vi "Layer1_ReceiveResponse.vi"(8 "Error In":errorcluster, 10 "Close Port After?":bool=TRUE, 11 "Serial Port to Use (In)":refnum<visa-resource-name>="COM8") -> (0 "Error Out":errorcluster, 1 "Layer1 Payload":string, 2 "Layer 1 Valid Packet":bool, 3 "Serial Port to Use (out)":refnum<visa-resource-name>, 5 "Raw Rx byte array":u8[](array[numeric]), 7 "Raw Receive Buffer":string)   [LabVIEW 2012]
uses:
  Arduino_Serial_GlobalConstants.vi
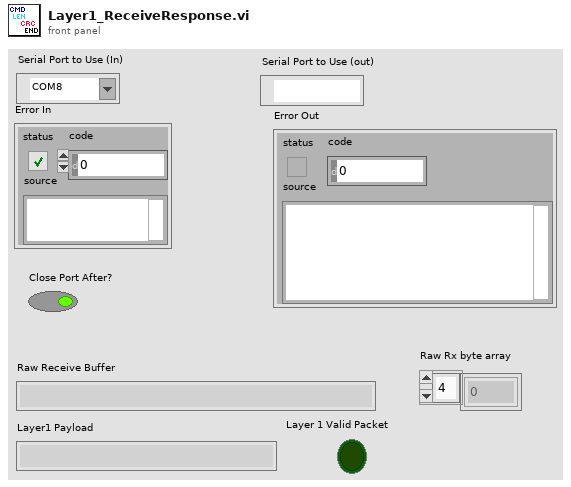
[diagram p1: front panel]
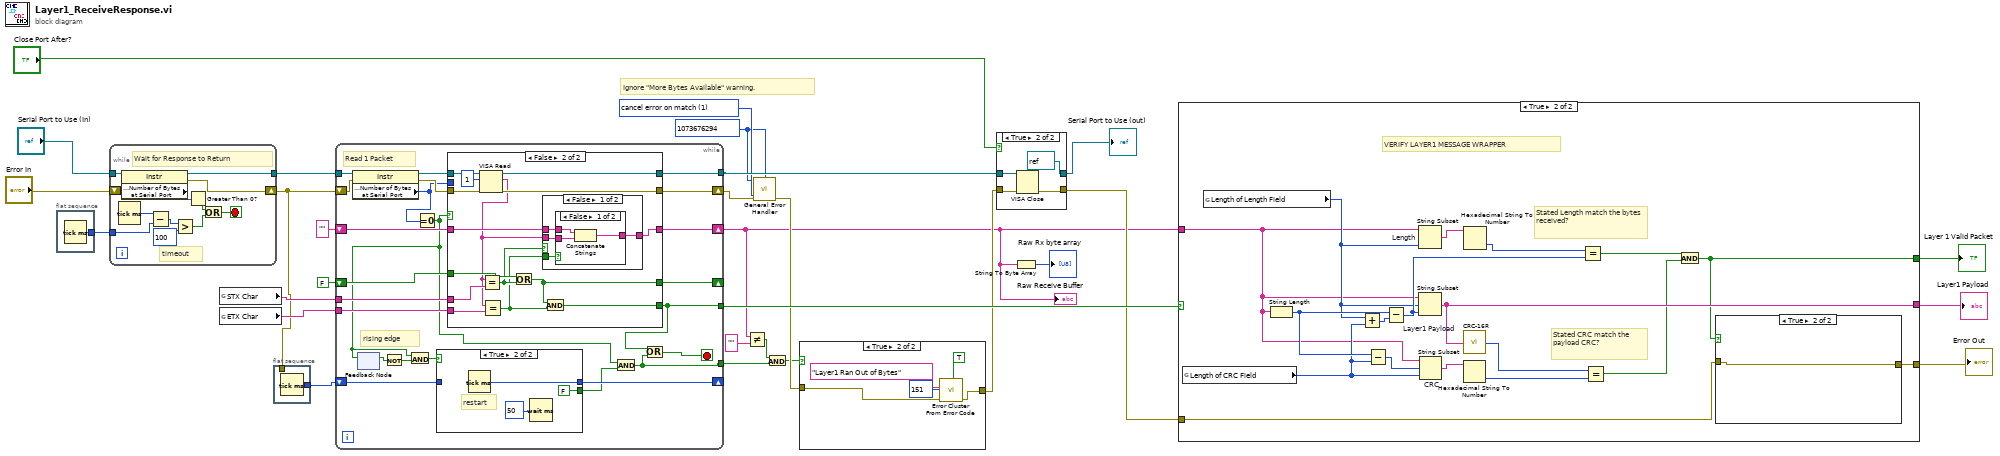
[diagram p0: block diagram]
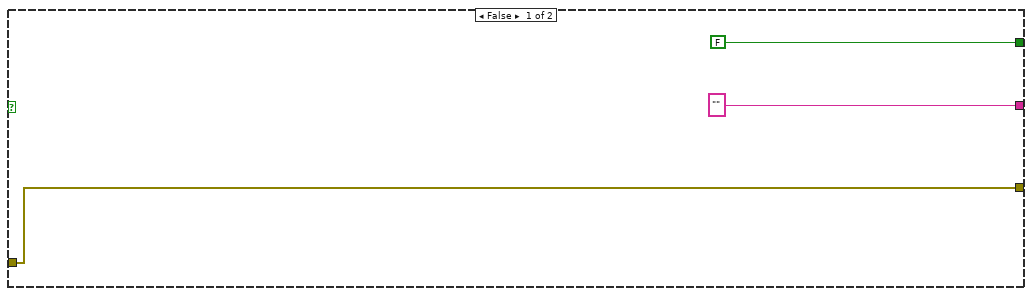
[diagram p4: hidden frame]
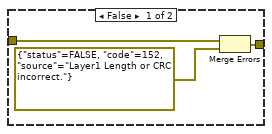
[diagram p5: hidden frame]
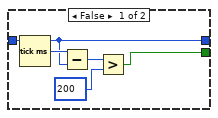
[diagram p6: hidden frame]
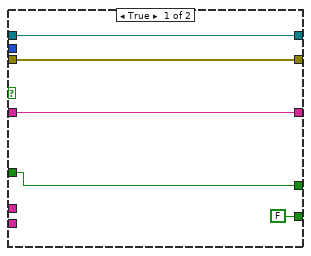
[diagram p7: hidden frame]
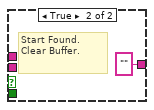
[diagram p9: hidden frame]
diagram:
  w8 = 1073676294 ("[exception code]")
  w9 = 1 items=["no exception", "cancel error on match", "set error on match"] ("[exception action] (none:0)")
  # "Ignore \"More Bytes Available\" warning."
  n1 = flat-sequence {
    tunnel: [w30] -> w22
    frame #0 {
      n2 = Tick Count (ms)() -> (millisecond timer value=w30:u32)
    }
  }
  n3 = while {
    tunnel: "Serial Port to Use (In)" -> [w42]
    shift-right: [w32] -> w13
    shift-left: "Error In" -> [w41]
    tunnel: w22 -> [w39]
    tunnel: [w33] -> w28
    stop <- w34 stop-if-true
    # "Wait for Response to Return"
    # "timeout"
    n4 = Tick Count (ms)() -> (millisecond timer value=w40:u32)
    n5 = property class="Instr"(reference=w42, error in=w41) -> (reference out=w33:refnum<visa-resource-name>, error out=w32:errorcluster, "Serial Settings:Number of Bytes at Serial Port"=w31:u32)
    n6 = Subtract(x=w40, y=w39) -> (x-y=w38:u32)
    n7 = Greater?(x=w38, y=u32 100) -> (0:w36:bool)
    n8 = Greater Than 0?(x=w31) -> (x > 0?=w35:bool)
    n9 = Or(x=w35, y=w36) -> (x .or. y?=w34:bool)
  }
  n10 = global read "Arduino_Serial_GlobalConstants.vi" "STX Char"() -> (w24:string)
  n11 = global read "Arduino_Serial_GlobalConstants.vi" "ETX Char"() -> (w23:string)
  n12 = flat-sequence {
    tunnel: [w43] -> w14
    tunnel: w13 -> [_]
    frame #0 {
      n13 = Tick Count (ms)() -> (millisecond timer value=w43:u32)
    }
  }
  n14 = while {
    tunnel: w28 -> [w66]
    shift-right: [w63] -> w7
    shift-left: w13 -> [w65]
    tunnel: [w62] -> w26
    shift-right: [w61] -> w5
    shift-left: "" -> [w60]
    tunnel: w24 -> [w57]
    tunnel: w23 -> [w56]
    shift-right: [w49] -> _
    shift-left: w14 -> [w50]
    shift-right: [w55] -> _
    shift-left: FALSE -> [w54]
    tunnel: [w52] -> w17
    tunnel: [w51] -> w1
    stop <- w53 stop-if-true
    # "rising edge"
    # "Read 1 Packet"
    n15 = property class="Instr"(reference=w66, error in=w65) -> (reference out=w64:refnum<visa-resource-name>, error out=w59:errorcluster, "Serial Settings:Number of Bytes at Serial Port"=w58:u32)
    n16 = feedback #1() -> (w44:bool)  [unwired: 1 in]
    n17 = Not(x=w44) -> (.not. x?=w45:bool)
    n18 = Equal To 0?(x=w58) -> (x = 0?=w46:bool)
    n19 = feedback-in #1(w46) -> ()
    n20 = And(x=w46, y=w45) -> (x .and. y?=w47:bool)
    n21 = case shown="True" w47 {
      tunnel: [w68 w74] -> w49
      tunnel: [w69 FALSE] -> w48
      tunnel: w50 -> [w68 _]
      frame False {
        n22 = Tick Count (ms)() -> (millisecond timer value=w71:u32)
        n23 = Subtract(x=w71, y=w68) -> (x-y=w70:u32)
        n24 = Greater?(x=w70, y=u32 200) -> (0:w69:bool)
      }
      frame True {
        # "restart"
        n25 = Tick Count (ms)() -> (millisecond timer value=w74:u32)
        n26 = Wait (ms)(milliseconds to wait=u32 50) -> ()  [unwired: 1 out]
      }
    }
    n27 = case shown="False" w46 {
      tunnel: w64 -> [w79 w94]
      tunnel: w59 -> [w78 w93]
      tunnel: w58 -> [_ _]
      tunnel: [w78 w92] -> w63
      tunnel: [w79 w91] -> w62
      tunnel: [w77 w80] -> w61
      tunnel: w60 -> [w77 w83]
      tunnel: w57 -> [_ w89]
      tunnel: w56 -> [_ w88]
      tunnel: [w76 w87] -> w55
      tunnel: w54 -> [w76 w85]
      tunnel: [FALSE w86] -> w52
      frame True {
      }
      frame False {
        n28 = VISA Read(VISA resource name=w94, byte count=u32 1, error in (no error)=w93) -> (VISA resource name out=w91:refnum<visa-resource-name>, read buffer=w82:string, error out=w92:errorcluster)  [unwired: 1 out]
        n29 = Equal?(x=w82, y=w89) -> (x = y?=w84:bool)
        n30 = Equal?(x=w82, y=w88) -> (x = y?=w81:bool)
        n31 = Or(x=w85, y=w84) -> (x .or. y?=w87:bool)
        n32 = case shown="False" w84 {
          tunnel: [w95 ""] -> w80
          tunnel: w83 -> [w97 _]
          tunnel: w82 -> [w96 _]
          tunnel: w81 -> [w98 _]
          frame False {
            n33 = case shown="False" w98 {
              tunnel: w97 -> [w101 w102]
              tunnel: w96 -> [w100 _]
              tunnel: [w99 w102] -> w95
              frame False {
                n34 = Concatenate Strings(w101, w100) -> (w99:string)
              }
              frame True {
                # "End Byte.\nDon't add."
              }
            }
          }
          frame True {
            # "Start Found.\nClear Buffer."
          }
        }
        n35 = And(x=w87, y=w81) -> (x .and. y?=w86:bool)
      }
    }
    n36 = And(x=w46, y=w48) -> (x .and. y?=w51:bool)
    n37 = Or(x=w52, y=w51) -> (x .or. y?=w53:bool)
  }
  "Raw Receive Buffer" <- w5
  n38 = Not Equal?(x=w5, y="") -> (x != y?=w2:bool)
  n39 = call <vilib>:"General Error Handler.vi"("[error code] (0)"=w8, "error in (no error)"=w7, "[exception action] (none:0)"=w9, "[exception code]"=w8) -> ("error out"=w6:errorcluster)  [unwired: 7 in, 4 out]
  n40 = And(x=w2, y=w1) -> (x .and. y?=w3:bool)
  n41 = case shown="True" w3 {
    tunnel: w6 -> [w104 w107]
    tunnel: [w104 w108] -> w10
    frame False {
    }
    frame True {
      n42 = call <vilib>:"Error Cluster From Error Code.vi"("is warning? (False)"=TRUE, "error in (no error)"=w107, "error message (\"\")"="Layer1 Ran Out of Bytes" ("source"), "error code (0)"=151) -> ("error out"=w108:errorcluster)  [unwired: 5 in]
    }
  }
  n43 = case shown="True" "Close Port After?" {
    tunnel: w10 -> [w111 w115]
    tunnel: w26 -> [w110 w114]
    tunnel: [w111 w113] -> w12
    tunnel: [w110 refnum<visa-resource-name> refnum ("VISA resource")] -> w15
    frame False {
    }
    frame True {
      n44 = VISA Close(VISA resource name=w114, error in (no error)=w115) -> (error out=w113:errorcluster)
    }
  }
  "Serial Port to Use (out)" <- w15
  n45 = String To Byte Array(string=w5) -> (unsigned byte array=→"Raw Rx byte array":u8[])
  n46 = case shown="True" w17 {
    tunnel: ["" w127] -> w21
    tunnel: [FALSE w119] -> w20
    tunnel: w5 -> [_ w122]
    tunnel: w12 -> [w116 w121]
    tunnel: [w116 w120] -> w11
    frame False {
    }
    frame True {
      # "VERIFY LAYER1 MESSAGE WRAPPER"
      # "Stated CRC match the payload CRC?"
      # "Stated Length match the bytes received?"
      n47 = global read "Arduino_Serial_GlobalConstants.vi" "Length of CRC Field"() -> (w123:i32)
      n48 = global read "Arduino_Serial_GlobalConstants.vi" "Length of Length Field"() -> (w124:i32)
      n49 = String Length(string=w122) -> (length=w132:i32)
      n50 = Add(x=w124, y=w123) -> (x+y=w131:i32)
      n51 = Subtract(x=w132, y=w123) -> (x-y=w133:i32)
      n52 = Subtract(x=w132, y=w131) -> (x-y=w128:i32)
      n53 = String Subset "Length"(string=w122, length (rest)=w124) -> (substring=w136:string)  [unwired: 1 in]
      n54 = String Subset "Layer1 Payload"(string=w122, offset (0)=w124, length (rest)=w128) -> (substring=w127:string)
      n55 = String Subset "CRC"(string=w122, offset (0)=w133, length (rest)=w123) -> (substring=w134:string)
      n56 = call <instrlib>:"CRC-16R.vi"("String"=w127) -> ("Checksum"=w130:u16)  [unwired: 2 out]
      n57 = Hexadecimal String To Number(string=w134) -> (number=w129:u32)  [unwired: 2 in, 1 out]
      n58 = Hexadecimal String To Number(string=w136) -> (number=w135:u32)  [unwired: 2 in, 1 out]
      n59 = Equal?(x=w135, y=w128) -> (x = y?=w126:bool)
      n60 = Equal?(x=w130, y=w129) -> (x = y?=w125:bool)
      n61 = And(x=w126, y=w125) -> (x .and. y?=w119:bool)
      n62 = case shown="True" w119 {
        tunnel: w121 -> [w138 w140]
        tunnel: [w139 w140] -> w120
        frame False {
          n63 = Merge Errors(w138, errorcluster {"status"=FALSE, "code"=152, "source"="Layer1 Length or CRC incorrect."} ("error in")) -> (w139:errorcluster)
        }
        frame True {
        }
      }
    }
  }
  "Layer 1 Valid Packet" <- w20
  "Layer1 Payload" <- w21
  "Error Out" <- w11
